vi "OpenExcel.vi"(8 "error in (no error)":errorcluster, 10 "name or relative path":string="SPR.csv") -> (0 "error out":errorcluster, 3 "all rows":string[](array[string]), 5 "appended path":path)   [LabVIEW 2011]
uses:
  <vilib>/Utility/file.llb/Read From Spreadsheet File (string).vi
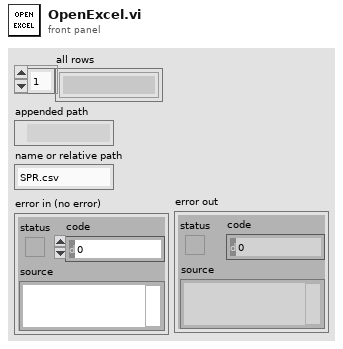
[diagram p1: front panel]
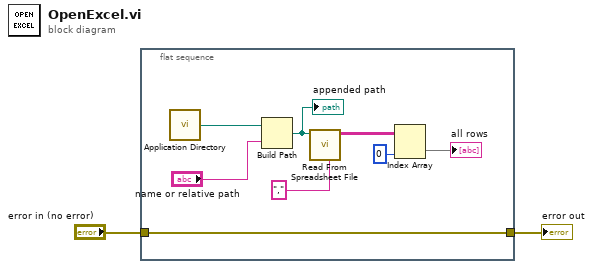
[diagram p0: block diagram]
diagram:
  n1 = flat-sequence {
    tunnel: "error in (no error)" -> [w4]
    tunnel: [w4] -> w1
    frame #0 {
      n2 = call <vilib>:"Application Directory.vi"() -> ("Application Directory"=w3:path)
      n3 = Build Path(base path=w3, name or relative path="name or relative path") -> (appended path=w10:path)
      "appended path" <- w10
      n4 = call-poly <vilib>:"Read From Spreadsheet File.vi"("delimiter (\\t)"="," ("delimiter (\\t)"), "file path (dialog if empty)"=w10) -> ("all rows"=w8:string[][])  [unwired: 5 in, 4 out]
      n5 = Index Array(array=w8, index (col)=0 ("disabled index (col)")) -> (element=→"all rows":string[])  [unwired: 1 in]
    }
  }
  "error out" <- w1
